vi "catch position translate.vi"(11 "main-national data":T1) -> (1 "output position":cluster{"horizontal":i32, "vertical":i32}[](array[cluster]), 3 "output cluster":T1)   [LabVIEW 2019]
uses:
  ctl/main data-national.ctl
  ctl/position set.ctl
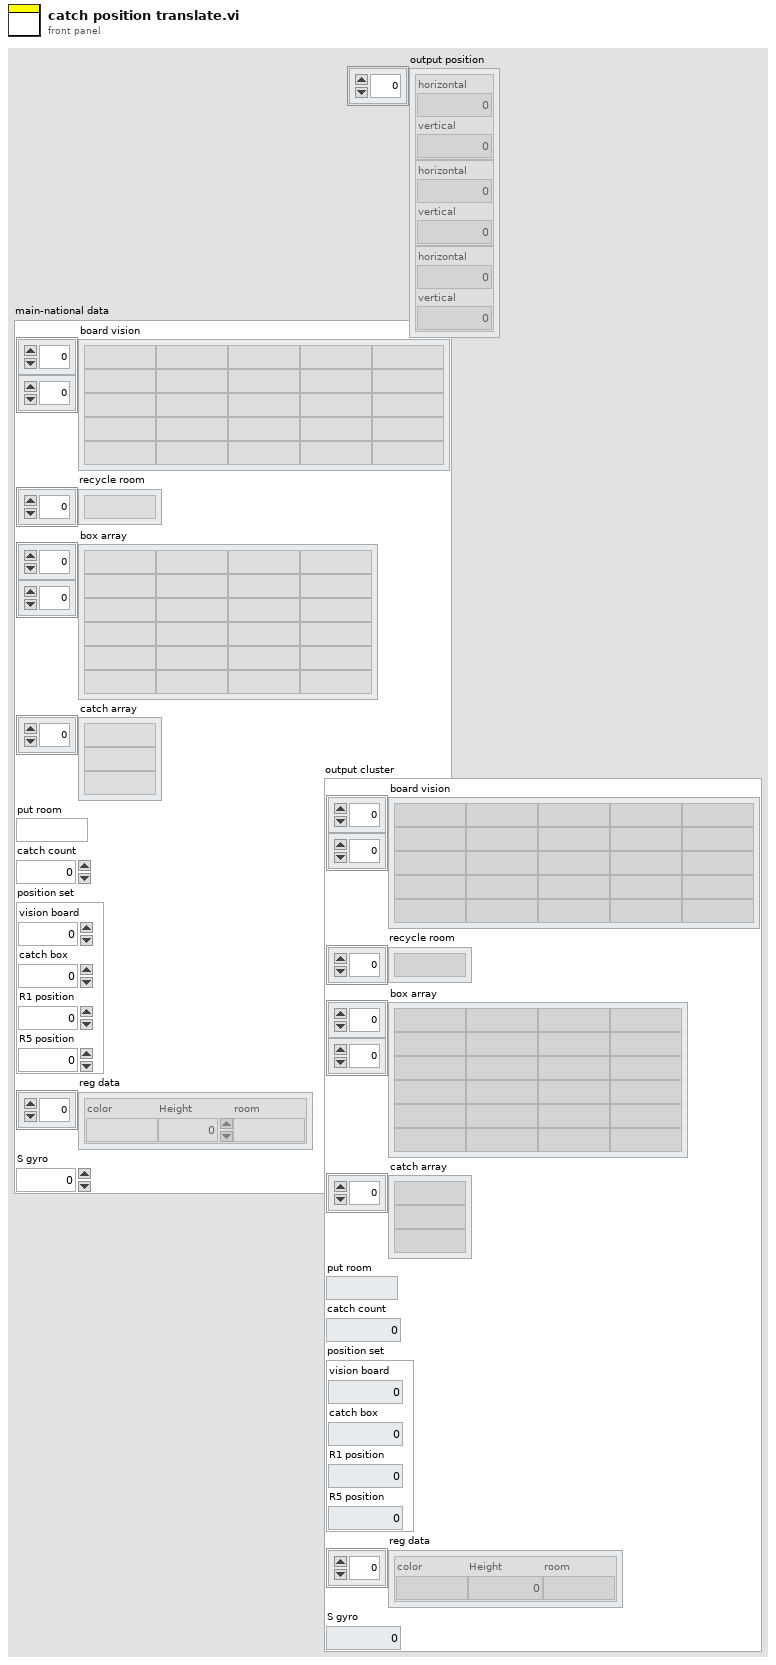
[diagram p1: front panel]
types:
  T1 = typedef "main data-national.ctl" = cluster{"board vision":string[][], "recycle room":string[], "box array":string[][], "catch array":string[], "put room":string, "catch count":dbl, "position set":T2, "reg data":cluster{"color":string, "Height":i32, "room":string}[], "S gyro":dbl}
  T2 = typedef "position set.ctl" = cluster{"vision board":dbl, "catch box":dbl, "R1 position":dbl, "R5 position":dbl}
  T3 = cluster{"color":string, "Height":i32, "room":string}[]
  T4 = cluster{"index of element":i32, "index of element":i32}
  T5 = cluster{"index of element":i32, "index of element":i32}[]
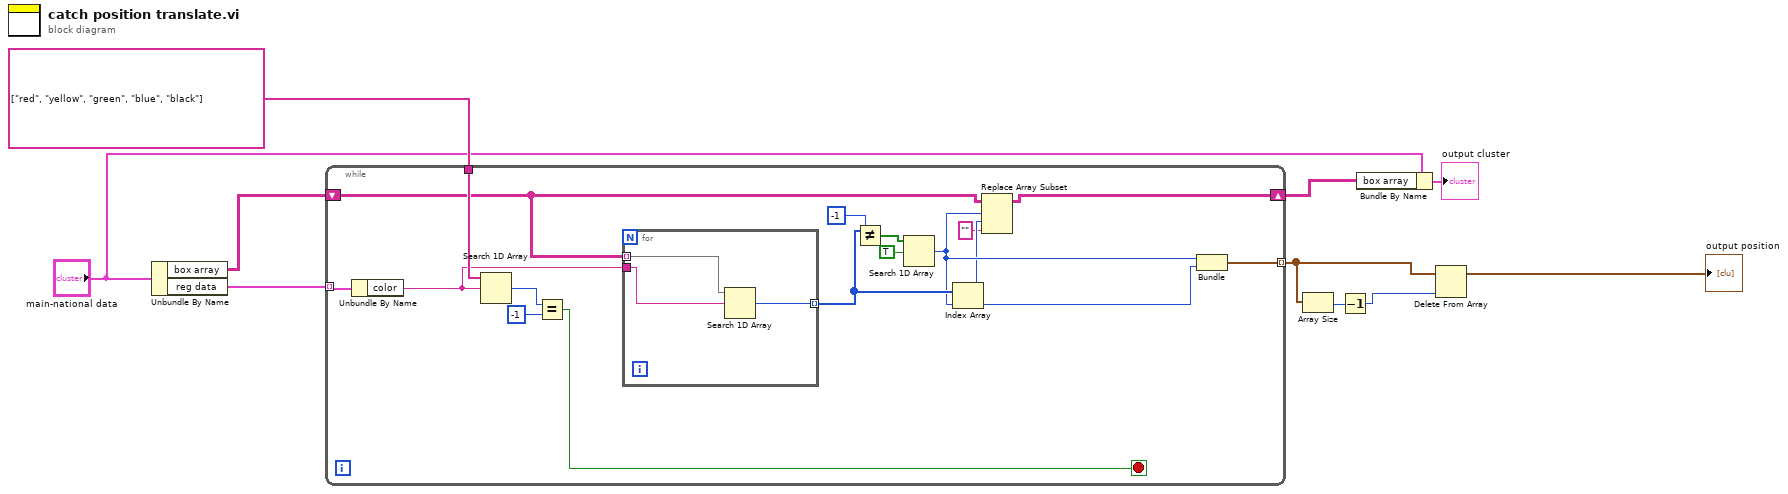
[diagram p0: block diagram]
diagram:
  n1 = Unbundle By Name("main-national data") -> ("box array"=w8:string[][], "reg data"=w10:T3)
  n2 = while {
    tunnel: w10 -> [w22] mode=indexing
    tunnel: string[] ["red", "yellow", "green", "blue", "black"] -> [w26]
    tunnel: [w17] -> w6 mode=indexing
    shift-right: [w12] -> w2
    shift-left: w8 -> [w16]
    stop <- w23 stop-if-true
    n3 = Unbundle By Name(w22) -> ("color"=w11:string)
    n4 = Search 1D Array(1D array=w26, element=w11) -> (index of element=w25:i32)  [unwired: 1 in]
    n5 = Equal?(x=w25, y=-1) -> (x = y?=w23:bool)
    n6 = for {
      tunnel: w11 -> [w29]
      tunnel: w16 -> [w28] mode=indexing
      tunnel: [w27] -> w18 mode=indexing
      n7 = Search 1D Array(1D array=w28, element=w29) -> (index of element=w27:i32)  [unwired: 1 in]
    }
    n8 = Not Equal?(x=w18, y=-1) -> (x != y?=w20:bool[])
    n9 = Search 1D Array(1D array=w20, element=TRUE) -> (index of element=w15:i32)  [unwired: 1 in]
    n10 = Index Array(array=w18, index=w15) -> (element=w14:i32)
    n11 = Replace Array Subset(array=w16, new element="" ("new element/subarray"), index (row)=w15, index (col)=w14) -> (w12:string[][])
    n12 = Bundle("index of element"=w15, "index of element"=w14) -> (w17:T4)  [unwired: 1 in]
  }
  n13 = Array Size(array=w6) -> (size(s)=w5:i32)
  n14 = Decrement(x=w5) -> (x-1=w4:i32)
  n15 = Bundle By Name(cluster="main-national data", "box array"=w2) -> (→"output cluster":T1)
  n16 = Delete From Array(array=w6, index=w4) -> (array with subset deleted=→"output position":T5)  [unwired: 1 in, 1 out]
